vi "Mvi-ImageData2Bytes.vi"() -> (0 "ErrOut":errorcluster)   [LabVIEW 2014]
doc: "Use this template to build a VI to use as a subVI."
panel:
  out "Image":T1(plugin-control)
  in  "ErrIn":errorcluster
  # "Input Parameters"
  # "Output Parameters"
  # "VI Description:\nThis VI is .."
  # ":: MVi Framework V1.0 ::\nAuthor:Gaoke Yang\nEmail: gaoke.yang@yahoo.com\nWeb: www.mvicontrol.com\nCopyright (C) 2015, MVI Technologies All Rights Reserved"
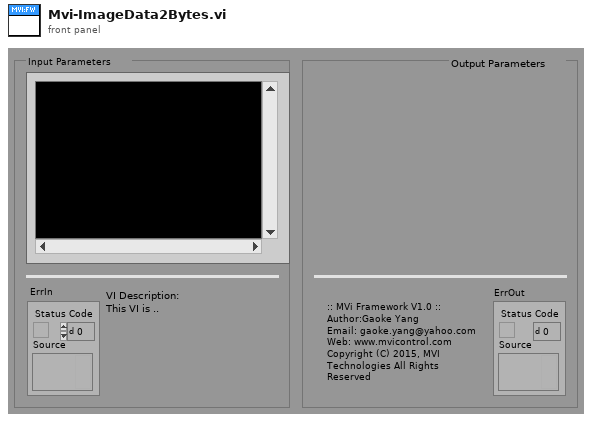
[diagram p1: front panel]
types:
  T1 = typedef "IMAQ Image.ctl" = refnum<image>
  T2 = enum16{"big-endian, network order", "native, host order", "little-endian"}
  T3 = typedef "Image Type" = u32
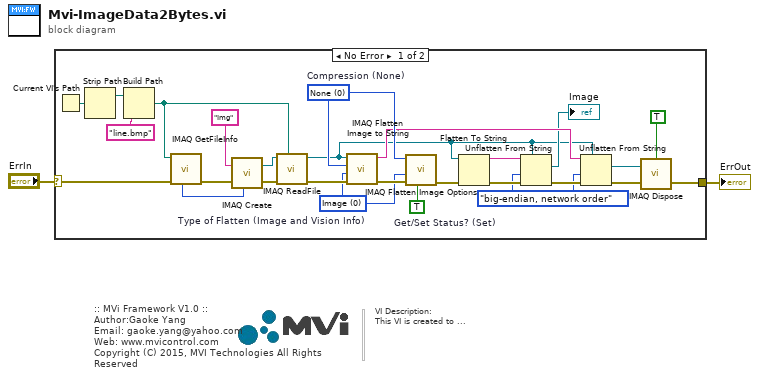
[diagram p0: block diagram]
diagram:
  # "VI Description:\nThis VI is created to ..."
  # ":: MVi Framework V1.0 ::\nAuthor:Gaoke Yang\nEmail: gaoke.yang@yahoo.com\nWeb: www.mvicontrol.com\nCopyright (C) 2015, MVI Technologies All Rights Reserved"
  n1 = case shown="No Error" "ErrIn" {
    selector: "ErrIn" -> [w22 w30]
    tunnel: [w4 w30] -> w2
    frame No Error {
      w7 = T2."big-endian, network order" ("byte order (0:big-endian, network order)")
      w16 = 0 items=["Image", "Image and Vision Info", "Reference to Image"]  # Type of Flatten (Image and Vision Info)
      w17 = 0 items=["None", "JPEG", "PACKED BINARY"]  # Compression (None)
      w20 = TRUE  # Get/Set Status? (Set)
      n2 = Current VI's Path() -> (path=w24:path)
      n3 = Strip Path(path=w24) -> (stripped path=w23:path)  [unwired: 1 out]
      n4 = Build Path(base path=w23, name or relative path="line.bmp") -> (appended path=w14:path)
      n5 = call "IMAQ GetFileInfo"("error in (no error)"=w22, "File Path"=w14) -> ("error out"=w27:errorcluster, "Image Type"=w26:T3)  [unwired: 3 in, 5 out]
      n6 = call "IMAQ Create"("Image Name"="Img", "Image Type"=w26, "error in (no error)"=w27) -> ("New Image"=w28:T1, "error out"=w21:errorcluster)  [unwired: 2 in]
      n7 = call "IMAQ ReadFile"("File Path"=w14, "error in (no error)"=w21, "Image"=w28) -> ("error out"=w19:errorcluster, "Image Out"=w8:T1)  [unwired: 4 in, 3 out]
      n8 = call "IMAQ Flatten Image to String"("error in (no error)"=w19, "Type of Flatten (Image and Vision Info)"=w16, "Compression (None)"=w17, "Image"=w8) -> ("error out"=w18:errorcluster, "Data String"=w11:string)  [unwired: 6 in]
      n9 = call "IMAQ Flatten Image Options"("Get/Set Status? (Set)"=w20, "error in (no error)"=w18, "Type of Flatten (Image and Vision Info)"=w16, "Compression (None)"=w17) -> ("error out"=w15:errorcluster)  [unwired: 4 in, 3 out]
      n10 = Flatten To String(anything=w8, error in (no error)=w15) -> (data string=w10:string, error out=w13:errorcluster)  [unwired: 2 in, 1 out]
      n11 = Unflatten From String(type=w8, binary string=w10, byte order (0:big-endian, network order)=w7, error in (no error)=w13) -> (value=→"Image":T1, error out=w12:errorcluster)  [unwired: 1 in, 1 out]
      n12 = Unflatten From String(type=w8, binary string=w11, byte order (0:big-endian, network order)=w7, error in (no error)=w12) -> (value=w6:T1, error out=w5:errorcluster)  [unwired: 1 in, 1 out]
      n13 = call "IMAQ Dispose"("All Images? (No)"=TRUE, "Image"=w6, "error in (no error)"=w5) -> ("error out"=w4:errorcluster)  [unwired: 3 in]
    }
    frame Error {
    }
  }
  "ErrOut" <- w2
